vi "USART_send_data.vi"(8 "error in":errorcluster, 10 "Coordinates":u32[](array[numeric]), 11 "VISA resource name in":refnum<visa-resource-name>) -> (0 "error out":errorcluster, 3 "VISA resource name out":refnum<visa-resource-name>)   [LabVIEW 2019]
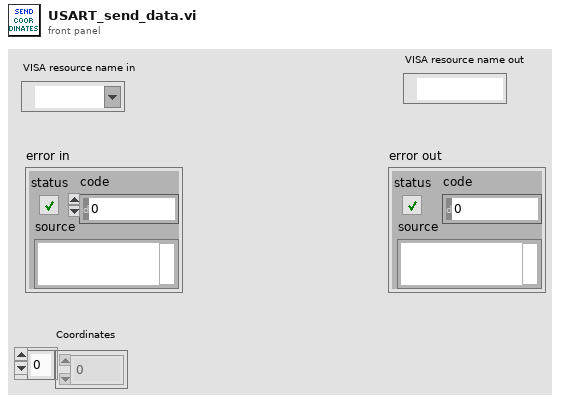
[diagram p1: front panel]
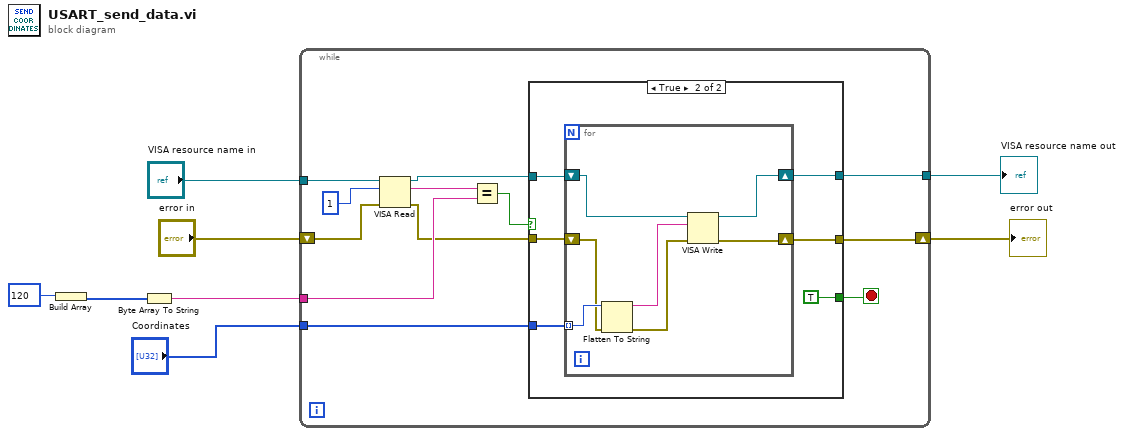
[diagram p0: block diagram]
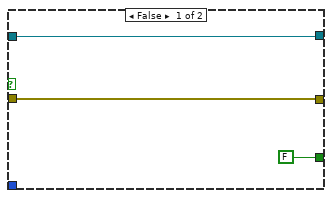
[diagram p2: hidden frame]
diagram:
  n1 = Build Array "Build Array"(120) -> (w6:i32[])
  n2 = Byte Array To String(unsigned byte array=w6) -> (string=w5:string)
  n3 = while {
    tunnel: "VISA resource name in" -> [w20]
    tunnel: w5 -> [w18]
    tunnel: "Coordinates" -> [w16]
    tunnel: [w12] -> w1
    shift-right: [w10] -> w2
    shift-left: "error in" -> [w11]
    stop <- w14 stop-if-true
    n4 = VISA Read(VISA resource name=w20, byte count=u32 1, error in (no error)=w11) -> (VISA resource name out=w13:refnum<visa-resource-name>, read buffer=w19:string, error out=w15:errorcluster)  [unwired: 1 out]
    n5 = Equal?(x=w19, y=w18) -> (x = y?=w17:bool)
    n6 = case shown="True" w17 {
      tunnel: w16 -> [_ w29]
      tunnel: w15 -> [w22 w27]
      tunnel: [FALSE TRUE] -> w14
      tunnel: [w22 w26] -> w10
      tunnel: w13 -> [w21 w25]
      tunnel: [w21 w24] -> w12
      frame False {
      }
      frame True {
        n7 = for {
          tunnel: w29 -> [w34] mode=indexing
          shift-right: [w32] -> w26
          shift-left: w27 -> [w33]
          shift-right: [w30] -> w24
          shift-left: w25 -> [w31]
          n8 = Flatten To String(anything=w34, error in (no error)=w33) -> (data string=w35:string, error out=w36:errorcluster)  [unwired: 2 in, 1 out]
          n9 = VISA Write(VISA resource name=w31, write buffer=w35, error in (no error)=w36) -> (VISA resource name out=w30:refnum<visa-resource-name>, error out=w32:errorcluster)  [unwired: 1 out]
        }
      }
    }
  }
  "error out" <- w2
  "VISA resource name out" <- w1
